vi "print_label.vi"(6 "all_config_info":T1={"main_ini_file"={"SQL Driver"="", "SQL Server"="", "SQL Database"="", "SQL UID"="", "Reference table"="", "Reference history"="", "Archivisation CFG table"="", "Archivisation CFG history"="", "User table"="", "User history"="", "default language"="", "SCANNER COM port"=0, "SCANNER Baud rate"=0, "SCANNER Data bits"=0, "SCANNER Pairity"=enum."None", "SCANNER Stop bits"=10, "SCANNER Flow control"=0, "SCANNER Termination char"=0, "PRINTER PC port"=0, "PRINTER IP"="", "PRINTER port"=0, "PRINTER Keep alive timer [ms]"=0, "logout timeout [ms]"=0}, "SQL Password"="", "PRINTER Label"="", "PRINTER Template"="", "Last Label"="", "queue_refnums"={"MAIN_queue"=refnum, "SCANNER_queue"=refnum, "SCANNER_login"=refnum, "PRINTER_queue"=refnum}} {"main_ini_file"."SCANNER Flow control" items=["None"=0, "XON/XOFF"=1, "RTS/CTS"=2, "DTR/DSR"=4]; "main_ini_file"."SCANNER Stop bits" items=["1.0"=10, "1.5"=15, "2.0"=20]}, 8 "error_in":errorcluster, 10 "do_printing? (T)":bool=TRUE, 11 "label_fields":T4) -> (0 "error_out":errorcluster)   [LabVIEW 2019]
uses:
  PRINTER/DOCK_PRINTER_label_fields.ctl
  ini/typedef/DOCK_all_config_info.ctl
  ini/typedef/DOCK_main_ini_file.ctl
  queues/typedef/DOCK_queue_refnums.ctl
  queues/typedef/DOCK_MAIN_queue_element.ctl
  DOCK_MAIN_sequence_state.ctl
  queues/typedef/DOCK_SCANNER_queue_element.ctl
  SCANNER/DOCK_SCANNER_sequence_state.ctl
  queues/typedef/DOCK_PRINTER_queue_element.ctl
  PRINTER/DOCK_PRINTER_sequence_state.ctl
  FGV/config_info/FGV_DOCK_config_info.ctl
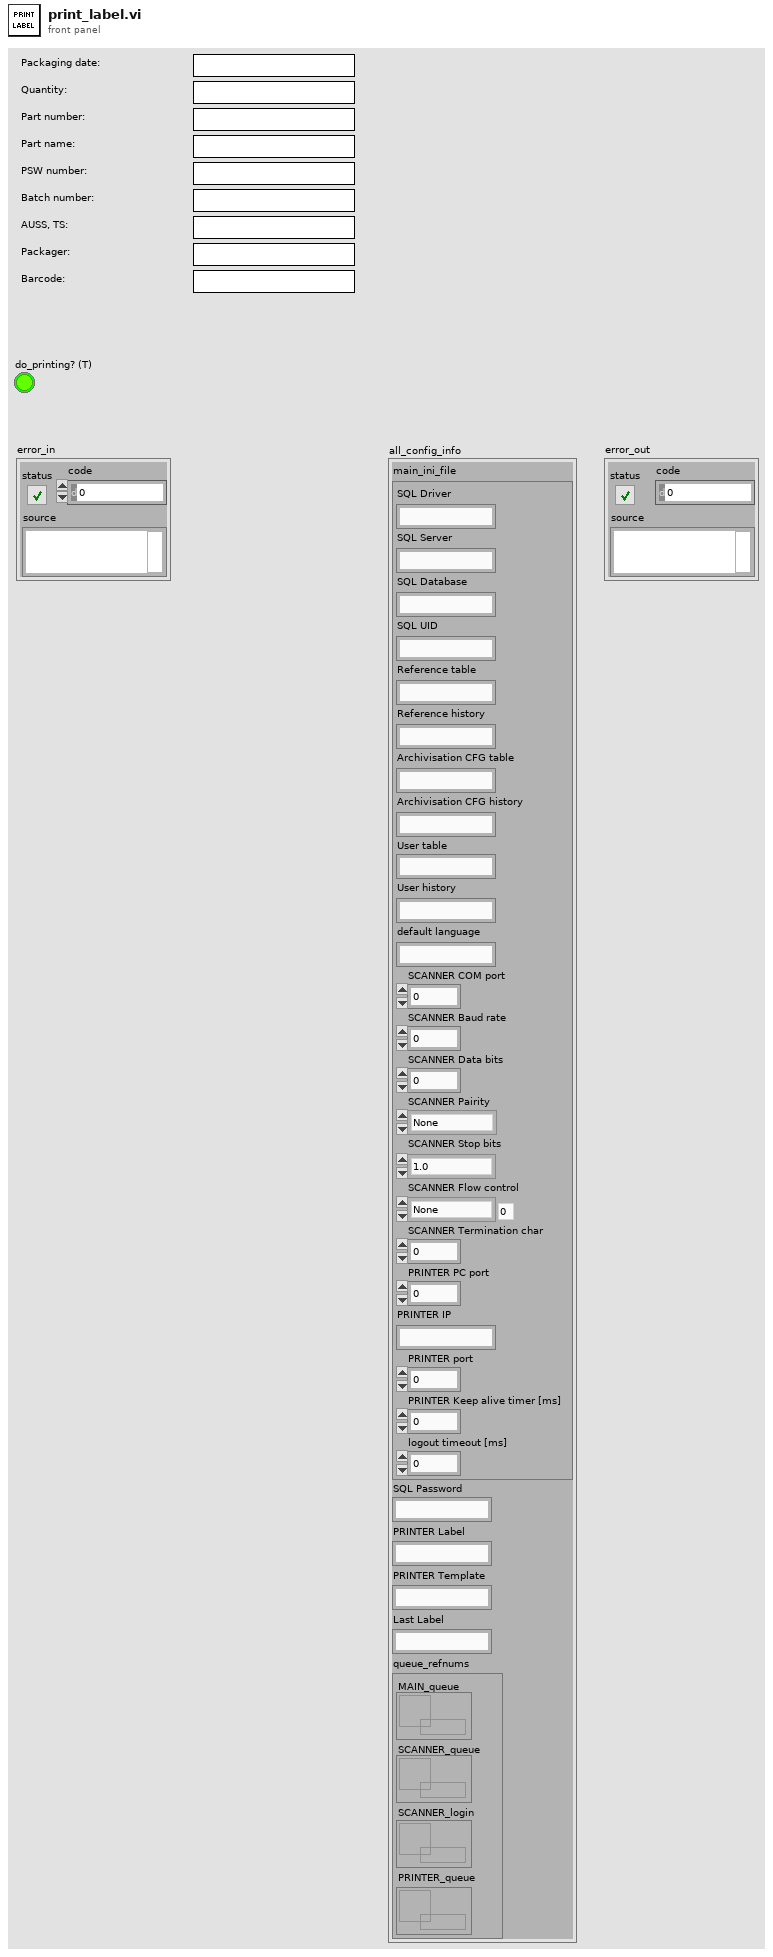
[diagram p1: front panel]
types:
  T1 = typedef "DOCK_all_config_info.ctl" = cluster{"main_ini_file":T2, "SQL Password":string, "PRINTER Label":string, "PRINTER Template":string, "Last Label":string, "queue_refnums":T3}
  T2 = typedef "DOCK_main_ini_file.ctl" = cluster{"SQL Driver":string, "SQL Server":string, "SQL Database":string, "SQL UID":string, "Reference table":string, "Reference history":string, "Archivisation CFG table":string, "Archivisation CFG history":string, "User table":string, "User history":string, "default language":string, "SCANNER COM port":u16, "SCANNER Baud rate":u32, "SCANNER Data bits":u16, "SCANNER Pairity":enum16{"None", "Odd", "Even", "Mark", "Space"}, "SCANNER Stop bits":u16, "SCANNER Flow control":u16, "SCANNER Termination char":u8, "PRINTER PC port":u16, "PRINTER IP":string, "PRINTER port":u16, "PRINTER Keep alive timer [ms]":i32, "logout timeout [ms]":i32}
  T3 = typedef "DOCK_queue_refnums.ctl" = cluster{"MAIN_queue":refnum<queue>, "SCANNER_queue":refnum<queue>, "SCANNER_login":refnum<queue>, "PRINTER_queue":refnum<queue>}
  T4 = typedef "DOCK_PRINTER_label_fields.ctl" = cluster{"packaging_date":string, "quantity":string, "part_number":string, "part_name":string, "PSW_number":string, "batch_number":string, "AUSS, TS":string, "packager":string, "barcode":string}
  T5 = typedef "FGV_DOCK_config_info.ctl" = enum16{"initialize", "set", "set_last_label", "get"}
  T6 = typedef "DOCK_PRINTER_queue_element.ctl" = cluster{"state":T7, "variable":variant}
  T7 = typedef "DOCK_PRINTER_sequence_state.ctl" = enum16{"initialize", "get_next_state", "send", "keep_alive", "error", "stop"}
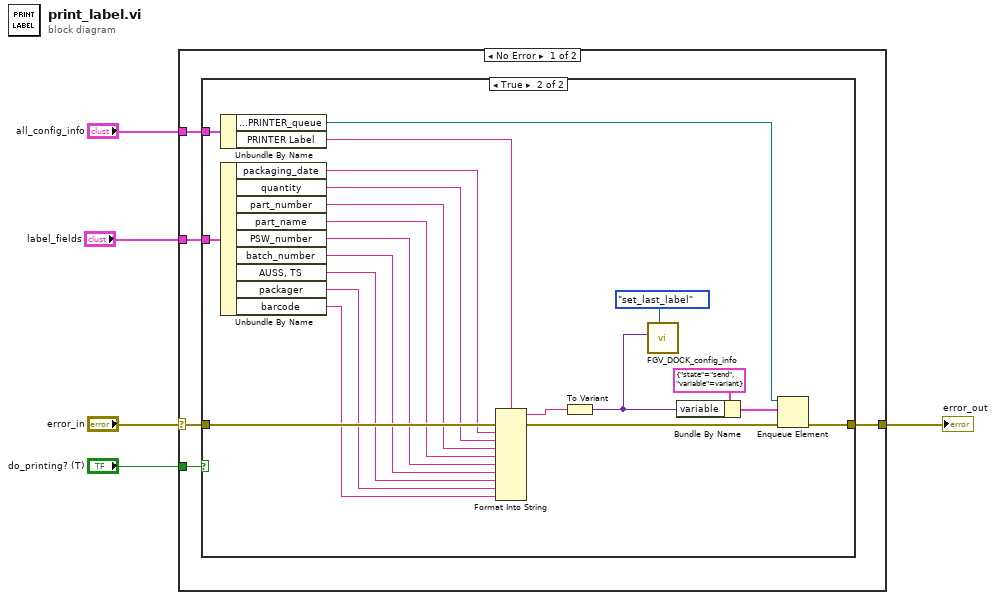
[diagram p0: block diagram]
diagram:
  n1 = case shown="No Error" "error_in" {
    selector: "error_in" -> [w8 w33]
    tunnel: [w7 w33] -> w4
    tunnel: "do_printing? (T)" -> [w10 _]
    tunnel: "all_config_info" -> [w9 _]
    tunnel: "label_fields" -> [w6 _]
    frame No Error {
      n2 = case shown="True" w10 {
        tunnel: w9 -> [_ w32]
        tunnel: w8 -> [w11 w30]
        tunnel: [w11 w18] -> w7
        tunnel: w6 -> [_ w29]
        frame False {
        }
        frame True {
          n3 = Unbundle By Name(w32) -> ("queue_refnums.PRINTER_queue"=w17:refnum<queue>, "PRINTER Label"=w31:string)
          n4 = Unbundle By Name(w29) -> ("packaging_date"=w28:string, "quantity"=w27:string, "part_number"=w26:string, "part_name"=w25:string, "PSW_number"=w24:string, "batch_number"=w23:string, "AUSS, TS"=w22:string, "packager"=w21:string, "barcode"=w20:string)
          n5 = Format Into String(format string=w31, error in=w30, w28, w27, w26, w25, w24, w23, w22, w21, w20) -> (resulting string=w14:string, error out=w19:errorcluster)  [unwired: 1 in]
          n6 = To Variant(anything=w14) -> (Variant=w12:variant)
          n7 = call "FGV_DOCK_config_info.vi"("options"=FGV_DOCK_config_info."set_last_label", "input"=w12) -> ()  [unwired: 8 in, 2 out]
          n8 = Bundle By Name(cluster=T6 {"state"=enum."send", "variable"=variant} ("element"), "variable"=w12) -> (w16:T6)
          n9 = Enqueue Element(queue=w17, element=w16, error in (no error)=w19) -> (error out=w18:errorcluster)  [unwired: 1 in, 2 out]
        }
      }
    }
    frame Error {
    }
  }
  "error_out" <- w4
